vi "Read Real Time Eye Measurements.vi"(8 "error in (no error)":errorcluster, 10 "Delay (5 s)":i32=5, 11 "VISA resource name":refnum<visa-resource-name>) -> (0 "error out":errorcluster, 1 "Eye Width":dbl, 2 "Eye Height":dbl, 3 "VISA resource name out":refnum<visa-resource-name>, 5 "UI Intervals Folded Into Real-Time Eye":i32)   [LabVIEW 2016, in "Agilent 2000 3000 X-Series.lvlib"]
doc: "Initiates data acquisition for the real-time eye analysis and fetches measurements after the specified.\n\n<b>Note:</b>\nThis VI is specific to the 6000-X Series oscilloscopes. These features are not available on other models."
uses:
  Agilent 2000 3000 X-Series.lvlib
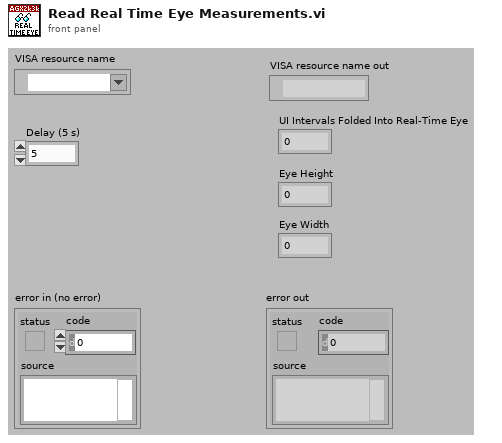
[diagram p1: front panel]
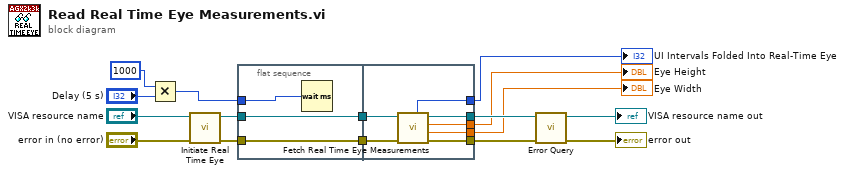
[diagram p0: block diagram]
diagram:
  n1 = Multiply(x=u32 1000, y="Delay (5 s)") -> (x*y=w11:u32)
  n2 = call "Initiate Real Time Eye.vi"("error in (no error)"="error in (no error)", "VISA resource name"="VISA resource name") -> ("error out"=w1:errorcluster, "VISA resource name out"=w3:refnum<visa-resource-name>)  [unwired: 8 in]
  n3 = flat-sequence {
    tunnel: w1 -> [w18]
    tunnel: w3 -> [w19]
    tunnel: [w19] -> w16
    tunnel: [w18] -> w15
    tunnel: w11 -> [w17]
    tunnel: w16 -> [w26]
    tunnel: w15 -> [w25]
    tunnel: [w21] -> w9
    tunnel: [w24] -> w8
    tunnel: [w22] -> w7
    tunnel: [w23] -> w6
    tunnel: [w20] -> w5
    frame #0 {
      n4 = Wait (ms)(milliseconds to wait=w17) -> ()  [unwired: 1 out]
    }
    frame #1 {
      n5 = call "Fetch Real Time Eye Measurements.vi"("error in (no error)"=w25, "VISA resource name"=w26) -> ("error out"=w24:errorcluster, "Eye Width"=w23:dbl, "Eye Height"=w22:dbl, "VISA resource name out"=w21:refnum<visa-resource-name>, "UI Intervals Folded Into Real-Time Eye"=w20:i32)  [unwired: 5 in]
    }
  }
  n6 = call "Error Query.vi"("error in (no error)"=w8, "VISA resource name"=w9) -> ("error out"=→"error out":errorcluster, "VISA resource name out"=→"VISA resource name out":refnum<visa-resource-name>)  [unwired: 6 in, 2 out]
  "Eye Height" <- w7
  "Eye Width" <- w6
  "UI Intervals Folded Into Real-Time Eye" <- w5
